vi "PDOTargetDevicePath.vi"(8 "error in (no error)":errorcluster, 9 "PDO Name":string, 10 "PDO Mapping":string, 11 "PDOTargetDevicePath":T1={"Pre_String"="ni.var.io", "Target Name"="RT PXI Target", "Master Name"="EtherCAT Master", "Device Name"="Device"}) -> (0 "error out":errorcluster, 3 "String":string)   [LabVIEW 2016, in "Motor Base.lvlib" / "Motor Base.lvclass"]
uses:
  Motor Base.lvclass
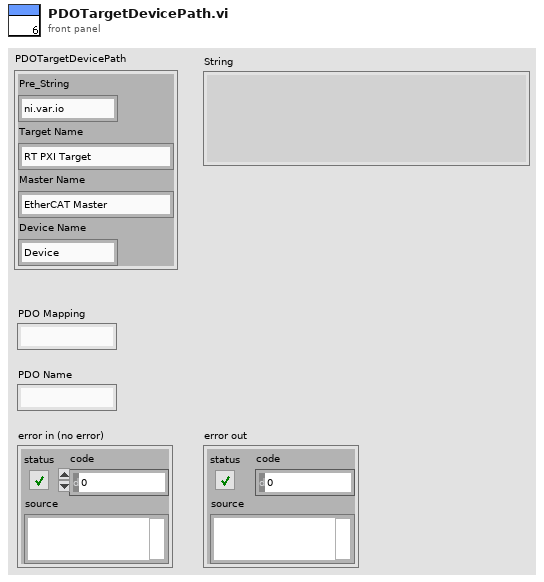
[diagram p1: front panel]
types:
  T1 = cluster{"Pre_String":string, "Target Name":string, "Master Name":string, "Device Name":string}
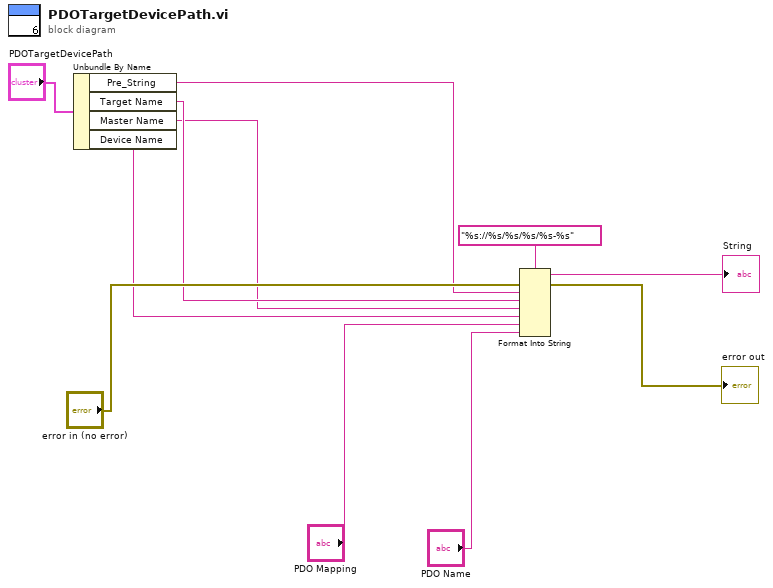
[diagram p0: block diagram]
diagram:
  n1 = Unbundle By Name("PDOTargetDevicePath") -> ("Pre_String"=w4:string, "Target Name"=w3:string, "Master Name"=w2:string, "Device Name"=w1:string)
  n2 = Format Into String(format string="%s://%s/%s/%s/%s-%s", error in="error in (no error)", w4, w3, w2, w1, "PDO Mapping", "PDO Name") -> (resulting string=→"String":string, error out=→"error out":errorcluster)  [unwired: 1 in]
